vi "BrokenLinkFGV.vi"(7 "Broken Chain FGV Action":T1, 8 "Error In":errorcluster, 10 "Broken?":bool, 11 "String":string) -> (0 "Error Out":errorcluster, 2 "VI broken? array":bool[](array[boolean]), 3 "VI names":string[](array[string]))   [LabVIEW 2017]
doc: "SciScan 1.2 160622\nThis FGV can be used to store the run status of VIs; and access its status at a later poinbt of time"
uses:
  Broken Chain FGV Command.ctl
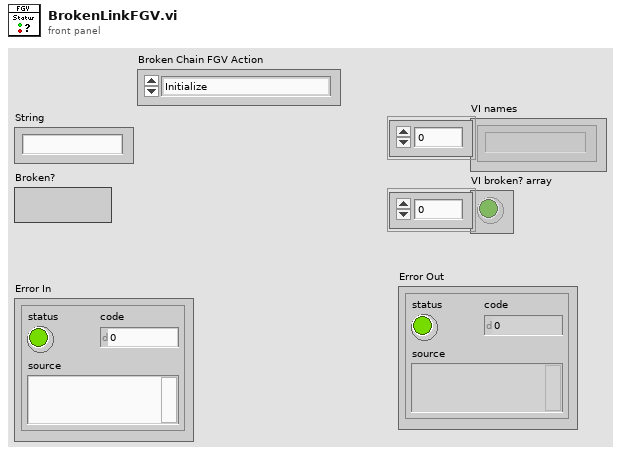
[diagram p1: front panel]
types:
  T1 = typedef "Broken Chain FGV Command.ctl" = enum16{"Initialize", "Update VI status", "Get All VI status"}
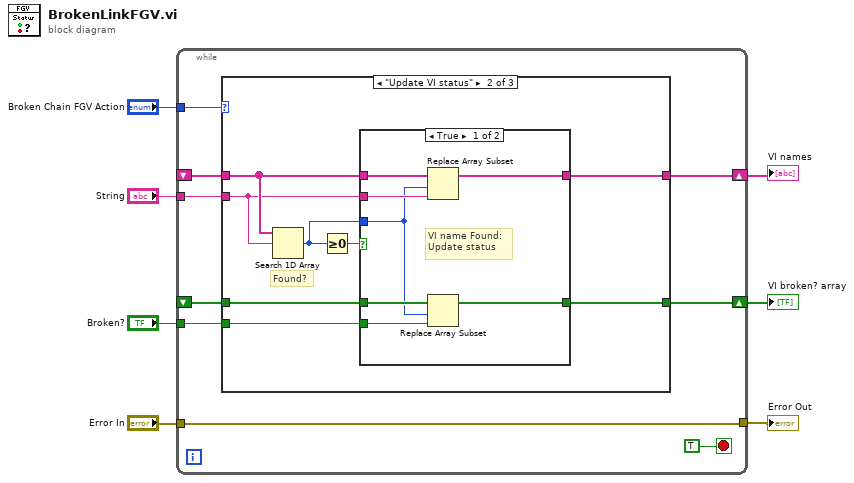
[diagram p0: block diagram]
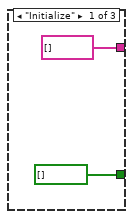
[diagram p2: hidden frame]
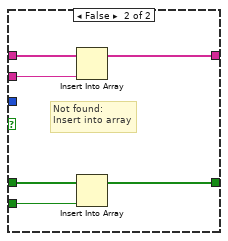
[diagram p3: hidden frame]
diagram:
  n1 = while {
    tunnel: "Broken Chain FGV Action" -> [w16]
    shift-right: [w15] -> w4
    shift-left: _ -> [w13]
    shift-right: [w12] -> w3
    shift-left: _ -> [w10]
    tunnel: "String" -> [w11]
    tunnel: "Broken?" -> [w9]
    tunnel: [w8] -> w1
    tunnel: "Error In" -> [w8]
    stop <- TRUE stop-if-true
    n2 = case shown="\"Update VI status\"" w16 {
      tunnel: [string[] [] w20 w41] -> w15
      tunnel: w13 -> [_ w25 w41]
      tunnel: [bool[] [] w21 w40] -> w12
      tunnel: w11 -> [_ w19 _]
      tunnel: w10 -> [_ w23 w40]
      tunnel: w9 -> [_ w22 _]
      frame "Initialize" {
      }
      frame "Update VI status" {
        # "Found?"
        n3 = Search 1D Array(1D array=w25, element=w19) -> (index of element=w24:i32)  [unwired: 1 in]
        n4 = Greater Or Equal To 0?(x=w24) -> (x >= 0?=w26:bool)
        n5 = case shown="True" w26 {
          tunnel: w25 -> [w33 w39]
          tunnel: w24 -> [w30 _]
          tunnel: w19 -> [w32 w38]
          tunnel: w23 -> [w31 w37]
          tunnel: w22 -> [w29 w36]
          tunnel: [w28 w35] -> w21
          tunnel: [w27 w34] -> w20
          frame True {
            # "VI name Found:\nUpdate status"
            n6 = Replace Array Subset(array=w33, new element=w32, index=w30) -> (w27:string[])
            n7 = Replace Array Subset(array=w31, new element=w29, index=w30) -> (w28:bool[])
          }
          frame False {
            # "Not found:\nInsert into array"
            n8 = Insert Into Array(array=w39, new element=w38) -> (w34:string[])  [unwired: 1 in]
            n9 = Insert Into Array(array=w37, new element=w36) -> (w35:bool[])  [unwired: 1 in]
          }
        }
      }
      frame "Get All VI status", Default {
      }
    }
  }
  "Error Out" <- w1
  "VI names" <- w4
  "VI broken? array" <- w3
